vi "Keyence LJ-X8000A Driver Test.vi"() -> ()   [LabVIEW 2020]
doc: "This example mainly shows the function of each VI.\nOn each button is the name of a VI. Click a button to perform that VI."
uses:
  Public/Clusters/Read Profile Req.ctl
  Public/Constants/Profile Pos.ctl
  Public/Clusters/Read Profile Rsp.ctl
  Public/Clusters/Profile Info.ctl
  Public/Clusters/Ethernet Config.ctl
  Public/Clusters/Read Batch Profile Rsp.ctl
  Public/Clusters/Read Batch Profile Req.ctl
  Public/Constants/Batch Pos.ctl
  Public/Constants/Setting Depth.ctl
  Public/Clusters/Target Setting.ctl
  Public/Constants/Setting Type.ctl
  Public/Constants/Init Setting Target.ctl
  KEYENCE LJ-X8000A.lvlib
panel:
  out "error out":errorcluster {"code" format="%.0x"}
  in  "tab2":T1(tab)
  in  "btnTrigger":bool
  in  "btnStartMeasure":bool
  in  "btnStopMeasure":bool
  in  "btnClearMemory":bool
  out "TRG_PASS":bool
  out "MEM_FULL":bool
  out "TRG_ERROR":bool
  in  "btnGetAttentionStatus":bool
  in  "State":bool
  in  "btnControlLaser":bool
  in  "btnResetTriggerError":bool
  in  "Read Req":T2={"Read Area"=enum."ACTIVE_BANK", "Profile Pos"=0, "Read Profile No."=0, "Read Profile Cnt"=1, "isErase"=FALSE} {"Profile Pos" items=["CURRENT", "OLDEST", "SPECIFY"]}
  in  "btnReadProfiles":bool
  in  "Data Size (0: Auto Size)":u32
  out "Profile Rsp":T4
  out "Profile Data":u32[](array[numeric])
  out "Profile Info":T5
  in  "btnReadBatchProfiles":bool
  out "Batch Profile Data":u32[](array[numeric])
  out "Batch Profile Info":T5
  out "Read Batch Profile Rsp":T6
  in  "Read Batch Profile Req":T7={"Read Area"=enum."ACTIVE_BANK", "Batch Pos"=0, "Read Batch No"=0, "Read Profile No."=0, "Read Profile Cnt"=1, "isErase"=FALSE} {"Batch Pos" items=["CURRENT"=0, "SPECIFY"=2, "COMMITED"=3, "NEWEST PROFILE"=4]}
  in  "Data Size (0: Auto Size) 2":u32
  in  "Read Req 2":T2={"Read Area"=enum."ACTIVE_BANK", "Profile Pos"=0, "Read Profile No."=0, "Read Profile Cnt"=1, "isErase"=FALSE} {"Profile Pos" items=["CURRENT", "OLDEST", "SPECIFY"]}
  in  "btnReadProfileArray":bool
  in  "Data Size (0: Auto Size) 4":u32
  out "Profile Rsp 2":T4
  out "Profile Info 2":T5
  out "Header Array":u32[][](array[numeric])
  out "Height Profile Array":dbl[][](array[numeric])
  out "Luminance Profile Array":u16[][](array[numeric])
  in  "btnReboot":bool
  in  "btnFactorySetting":bool
  in  "btnGetHeadTemperature":bool
  in  "btnGetSerialNo":bool
  out "Controller Serial No.":string
  out "Head Serial No.":string
  in  "btnGetSystemError":bool
  in  "Get Code Cnt":u8=1
  in  "btnGetTriggerAndPulseCnt":bool
  out "Trigger Count":u32
  out "Encoder Count":i32
  out "Error Code":u16[](array[numeric]) format="%04x"
  out "Sensor Temperature":i16
  out "Processor Temperature":i16
  out "Case Temperature":i16
  in  "btnClearSystemError":bool
  out "Error Cnt":u8
  in  "Cleared Error Code":u16 format="%04x"
  out "Memory Accessing":bool
  out "Memory Accessing":bool
  in  "Target Setting":T9={"Type"=16, "Category"=0, "Item"=2, "Target 1"=0, "Target 2"=0, "Target 3"=0, "Target 4"=0} {"Target 4" format="%.0x"; "Target 3" format="%.0x"; "Target 2" format="%.0x"; "Target 1" format="%.0x"; "Item" format="%.0x"; "Category" format="%.0x"; "Type" items=["ENVIRONMENT"=1, "COMMON MEASUREMENT"=2, "PROGRAM 0"=16, "PROGRAM 1"=17, "PROGRAM 2"=18, "PROGRAM 3"=19, "PROGRAM 4"=20, "PROGRAM 5"=21, "PROGRAM 6"=22, "PROGRAM 7"=23, "PROGRAM 8"=24, "PROGRAM 9"=25, "PROGRAM 10"=26, "PROGRAM 11"=27, "PROGRAM 12"=28, "PROGRAM 13"=29, "PROGRAM 14"=30, "PROGRAM 15"=31]}
  in  "Depth":T11=1 items=["WRITE AREA", "RUNNING AREA", "SAVE AREA"]
  in  "btnChangeProgram":bool
  in  "btnGetProgram":bool
  in  "Program No":u8
  out "Active Program No.":u8
  in  "Target Setting":T9={"Type"=16, "Category"=0, "Item"=2, "Target 1"=0, "Target 2"=0, "Target 3"=0, "Target 4"=0} {"Target 4" format="%.0x"; "Target 3" format="%.0x"; "Target 2" format="%.0x"; "Target 1" format="%.0x"; "Item" format="%.0x"; "Category" format="%.0x"; "Type" items=["ENVIRONMENT"=1, "COMMON MEASUREMENT"=2, "PROGRAM 0"=16, "PROGRAM 1"=17, "PROGRAM 2"=18, "PROGRAM 3"=19, "PROGRAM 4"=20, "PROGRAM 5"=21, "PROGRAM 6"=22, "PROGRAM 7"=23, "PROGRAM 8"=24, "PROGRAM 9"=25, "PROGRAM 10"=26, "PROGRAM 11"=27, "PROGRAM 12"=28, "PROGRAM 13"=29, "PROGRAM 14"=30, "PROGRAM 15"=31]}
  out "Setting Data":u8[](array[numeric])
  in  "Depth":T11=1 items=["WRITE AREA", "RUNNING AREA", "SAVE AREA"]
  in  "btnGetSetting":bool
  in  "Data Size":u32=4
  in  "btnSetSetting":bool
  in  "Setting Data":u8[](array[numeric])=[3, 0, 0, 0]
  out "Setting Error":u32 format="%.0x"
  out "Memory Accessing":bool
  in  "Depth":T11 items=["WRITE AREA", "RUNNING AREA", "SAVE AREA"]
  in  "btnInitializeSetting":bool
  in  "Target Program":T12 items=["PROGRAM 0", "PROGRAM 1", "PROGRAM 2", "PROGRAM 3", "PROGRAM 4", "PROGRAM 5", "PROGRAM 6", "PROGRAM 7", "PROGRAM 8", "PROGRAM 9", "PROGRAM 10", "PROGRAM 11", "PROGRAM 12", "PROGRAM 13", "PROGRAM 14", "PROGRAM 15"]
  in  "Depth":T11 items=["WRITE AREA", "RUNNING AREA", "SAVE AREA"]
  in  "btnReflectSetting":bool
  out "Setting Error":u32
  in  "btnUpdateWriteSettingArea":bool
  in  "Depth":T11 items=["WRITE AREA", "RUNNING AREA", "SAVE AREA"]
  in  "btnLogClear":bool
  in  "btnClose":bool
  out "Operation Result Log":string
  out "isConnecting":bool caption="Connecting"
  in  "Ethernet Config":T13={"IP Address"=[192, 168, 0, 1], "Port No"=24691}
  in  "btnInitialize":bool
  in  "stop":bool caption="’âŽ~"
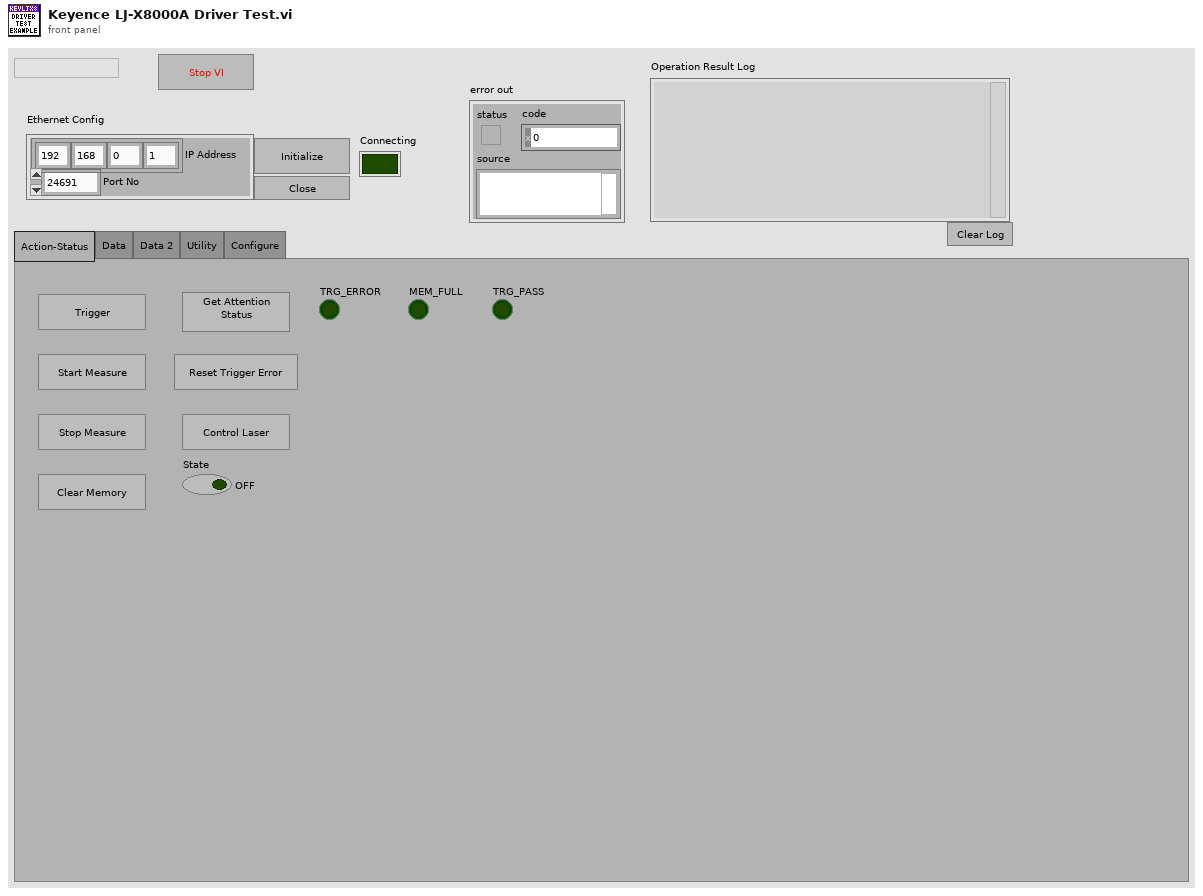
[diagram p1: front panel]
types:
  T1 = enum32{"Action-Status", "Data", "Data 2", "Utility", "Configure"}
  T2 = typedef "KEYENCE LJ-X8000A.lvlib/Read Profile Req.ctl" = cluster{"Read Area":enum8{"ACTIVE_BANK", "INACTIVE_BANK"}, "Profile Pos":T3, "Read Profile No.":u32, "Read Profile Cnt":u8, "isErase":bool}
  T3 = typedef "KEYENCE LJ-X8000A.lvlib/Profile Pos.ctl" = u8
  T4 = typedef "KEYENCE LJ-X8000A.lvlib/Read Profile Rsp.ctl" = cluster{"Current Profile No":u32, "Oldest Profile No":u32, "Read Top Profile No":u32, "Read Profile Cnt":u8}
  T5 = typedef "KEYENCE LJ-X8000A.lvlib/Profile Info.ctl" = cluster{"Profile Cnt":u8, "Luminance Output":bool, " Profile Data Point":u16, " X Start":i32, " X Pitch":i32}
  T6 = typedef "KEYENCE LJ-X8000A.lvlib/Read Batch Profile Rsp.ctl" = cluster{"Current Batch No":u32, "Current Batch Profile Cnt":u32, "Oldest Batch No":u32, "Oldest Batch Profile Cnt":u32, "Read Batch No":u32, "Read Batch Profile Cnt":u32, "Read Batch Top Profile No":u32, "Read Profile Cnt":u32, "Current Batch Commited":bool}
  T7 = typedef "KEYENCE LJ-X8000A.lvlib/Read Batch Profile Req.ctl" = cluster{"Read Area":enum8{"ACTIVE_BANK", "INACTIVE_BANK"}, "Batch Pos":T8, "Read Batch No":u32, "Read Profile No.":u32, "Read Profile Cnt":u8, "isErase":bool}
  T8 = typedef "KEYENCE LJ-X8000A.lvlib/Batch Pos.ctl" = u8
  T9 = typedef "KEYENCE LJ-X8000A.lvlib/Target Setting.ctl" = cluster{"Type":T10, "Category":u8, "Item":u8, "Target 1":u8, "Target 2":u8, "Target 3":u8, "Target 4":u8}
  T10 = typedef "KEYENCE LJ-X8000A.lvlib/Setting Type.ctl" = u8
  T11 = typedef "KEYENCE LJ-X8000A.lvlib/Setting Depth.ctl" = u8
  T12 = typedef "KEYENCE LJ-X8000A.lvlib/Init Setting Target.ctl" = u8
  T13 = typedef "KEYENCE LJ-X8000A.lvlib/Ethernet Config.ctl" = cluster{"IP Address":u8[], "Port No":u16}
  T14 = enum8{"Enabled", "Disabled", "Disabled and Grayed Out"}
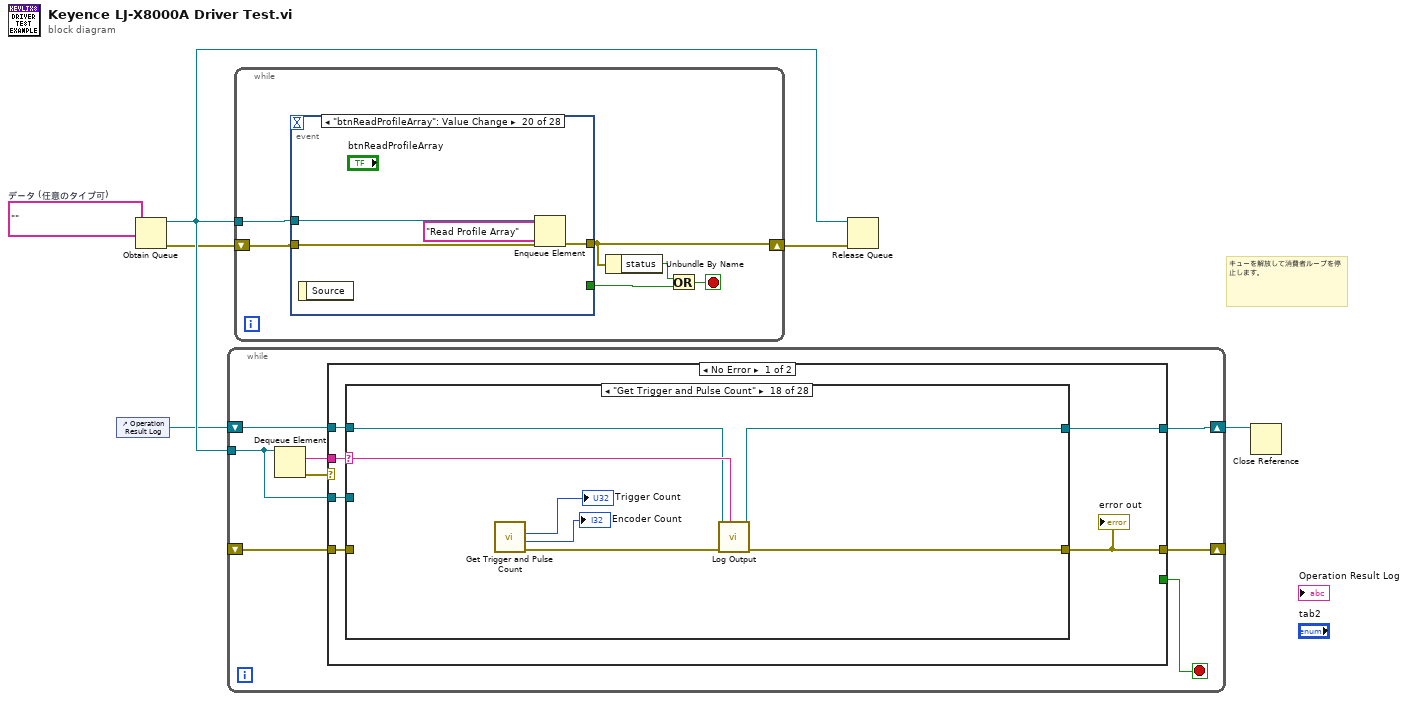
[diagram p0: block diagram]
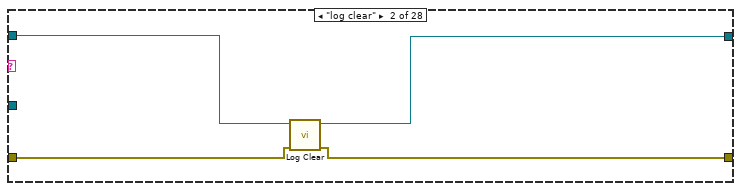
[diagram p3: hidden frame]
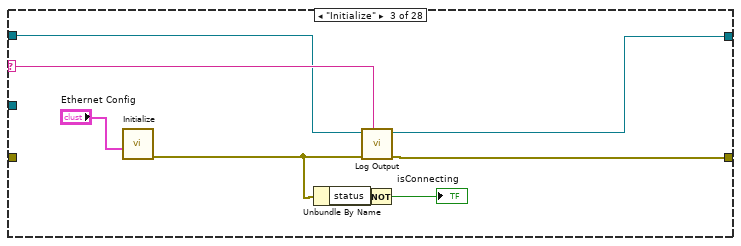
[diagram p4: hidden frame]
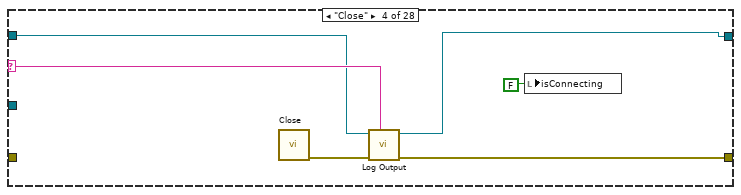
[diagram p5: hidden frame]
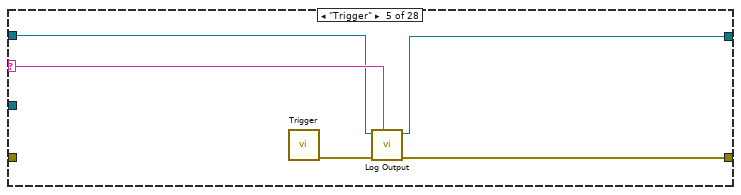
[diagram p6: hidden frame]
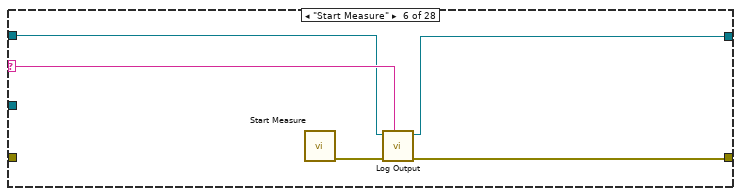
[diagram p7: hidden frame]
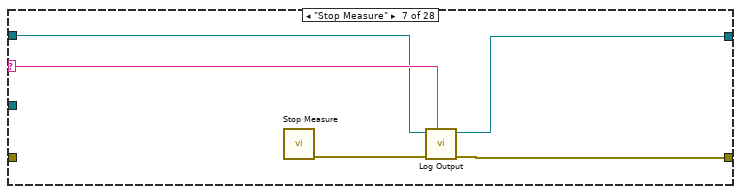
[diagram p8: hidden frame]
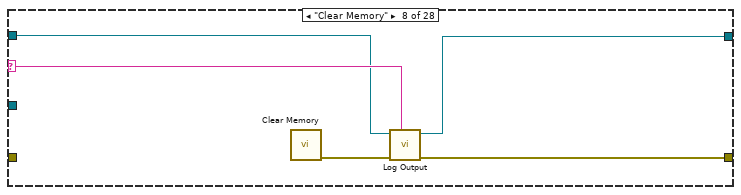
[diagram p9: hidden frame]
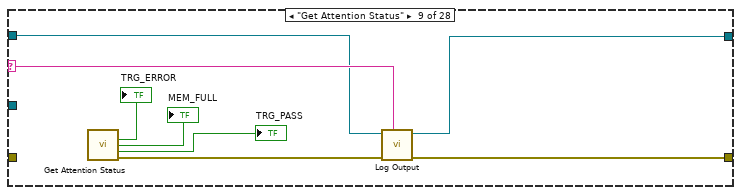
[diagram p10: hidden frame]
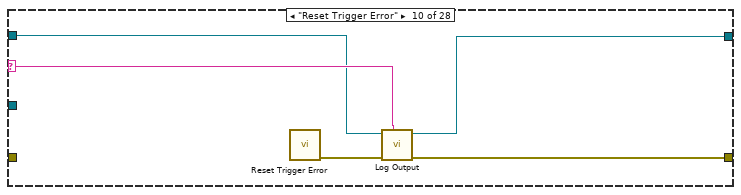
[diagram p11: hidden frame]
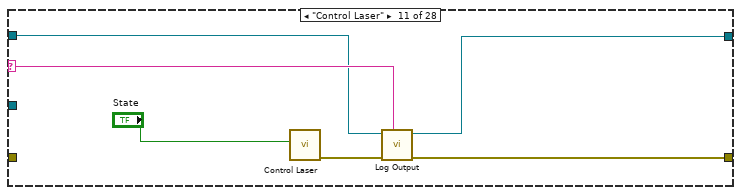
[diagram p12: hidden frame]
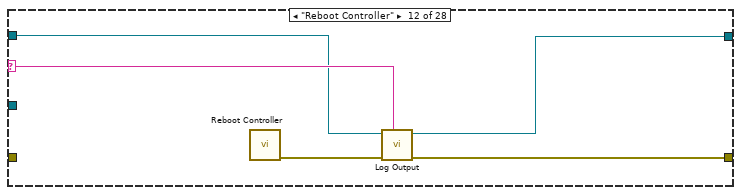
[diagram p13: hidden frame]
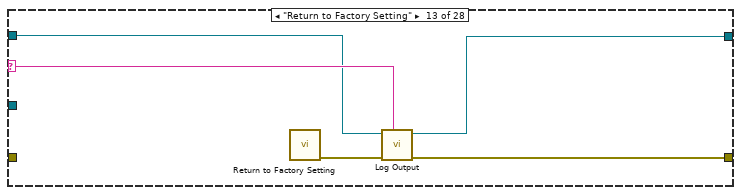
[diagram p14: hidden frame]
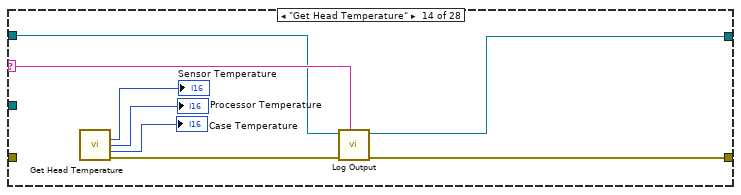
[diagram p15: hidden frame]
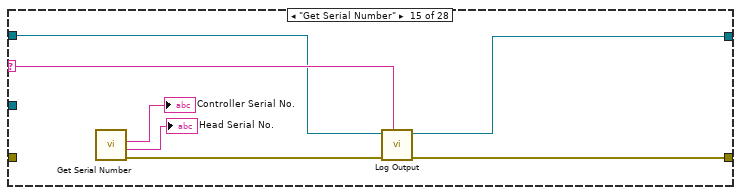
[diagram p16: hidden frame]
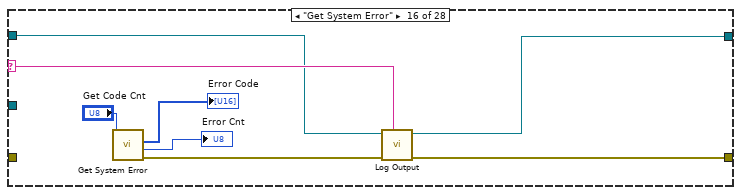
[diagram p17: hidden frame]
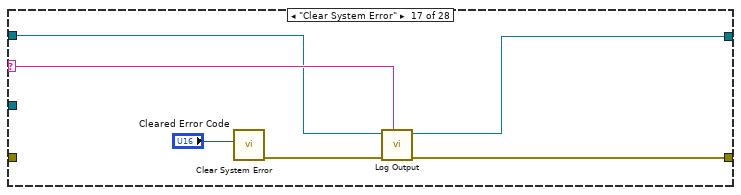
[diagram p18: hidden frame]
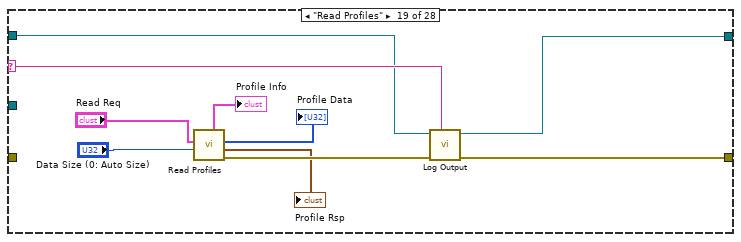
[diagram p19: hidden frame]
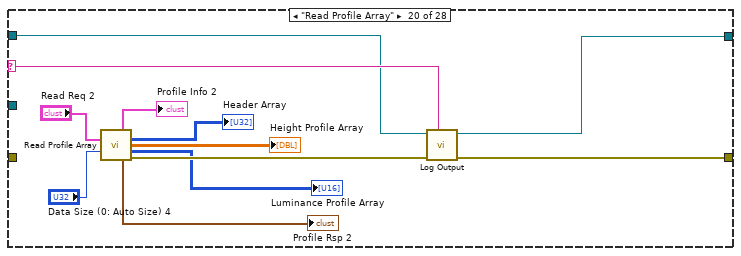
[diagram p20: hidden frame]
diagram:
  w6 = ""  # データ (任意のタイプ可)
  # "キューを解放して消費者ループを停止します。"
  n1 = control-ref of="Operation Result Log"() -> (w2:refnum<vi>)
  n2 = Obtain Queue(element data type=w6) -> (queue out=w5:refnum<queue>, error out=w3:errorcluster)  [unwired: 4 in, 1 out]
  n3 = while {
    tunnel: w5 -> [w10]
    shift-right: [w9] -> _
    shift-left: _ -> [w11]
    shift-right: [w7] -> w1
    shift-left: w2 -> [w8]
    stop <- w12 stop-if-true
    n4 = Dequeue Element(queue=w10) -> (element=w13:string, error out=w14:errorcluster)  [unwired: 2 in, 2 out]
    n5 = case shown="No Error" w14 {
      selector: w14 -> [_ w243]
      tunnel: w13 -> [w20 _]
      tunnel: [_ TRUE] -> w12
      tunnel: [w19 w243] -> w9
      tunnel: w11 -> [w18 _]
      tunnel: w10 -> [w17 _]
      tunnel: w8 -> [w15 w241]
      tunnel: [w16 w241] -> w7
      frame No Error {
        n6 = case shown="\"Get Trigger and Pulse Count\"" w20 {
          selector: w20 -> [_ _ w29 w37 w43 w48 w53 w58 w63 w71 w76 w82 w87 w92 w100 w107 w115 w121 w128 w146 w150 w160 w166 w172 w181 w203 w222 w237]
          tunnel: [w22 w24 w30 w38 w44 w49 w54 w59 w68 w73 w79 w84 w89 w97 w104 w112 w118 w125 w135 w147 w157 w163 w169 w178 w184 w201 w219 w240] -> w19
          tunnel: w18 -> [w22 w25 _ _ _ _ _ _ _ _ _ _ _ _ _ _ _ _ _ _ _ _ _ _ _ _ _ _]
          tunnel: w17 -> [_ _ _ _ _ _ _ _ _ _ _ _ _ _ _ _ _ _ _ _ _ _ _ _ _ _ _ _]
          tunnel: w15 -> [w21 w26 w28 w36 w42 w47 w52 w57 w62 w70 w75 w81 w86 w91 w99 w106 w114 w120 w127 w137 w149 w159 w165 w170 w180 w200 w218 w236]
          tunnel: [w21 w23 w27 w35 w41 w46 w51 w56 w61 w69 w74 w80 w85 w90 w98 w105 w113 w119 w126 w136 w148 w158 w164 w171 w179 w199 w217 w235] -> w16
          frame Default {
          }
          frame "log clear" {
            n7 = call "Log Clear.vi"("error in (no error)"=w25, "Result Log Reference"=w26) -> ("error out"=w24:errorcluster, "Result Log Reference Out"=w23:refnum<vi>)  [unwired: 8 in]
          }
          frame "Initialize" {
            n8 = call "Initialize.vi"("Ethernet Config"="Ethernet Config") -> ("error out"=w31:errorcluster)  [unwired: 9 in, 1 out]
            n9 = Unbundle By Name(w31) -> ("status"=w33:bool)
            n10 = call "Log Output.vi"("VI Name"=w29, "error in (no error)"=w31, "Result Log Reference"=w28) -> ("error out"=w30:errorcluster, "Result Log Reference Out"=w27:refnum<vi>)  [unwired: 6 in]
            n11 = Not(x=w33) -> (.not. x?=→"isConnecting":bool)
          }
          frame "Close" {
            n12 = call "Close.vi"() -> ("error out"=w39:errorcluster)  [unwired: 10 in, 1 out]
            n13 = call "Log Output.vi"("VI Name"=w37, "error in (no error)"=w39, "Result Log Reference"=w36) -> ("error out"=w38:errorcluster, "Result Log Reference Out"=w35:refnum<vi>)  [unwired: 6 in]
            n14 = local write "isConnecting"(FALSE ("isConnecting")) -> ()
          }
          frame "Trigger" {
            n15 = call "Trigger.vi"() -> ("error out"=w45:errorcluster)  [unwired: 10 in, 1 out]
            n16 = call "Log Output.vi"("VI Name"=w43, "error in (no error)"=w45, "Result Log Reference"=w42) -> ("error out"=w44:errorcluster, "Result Log Reference Out"=w41:refnum<vi>)  [unwired: 6 in]
          }
          frame "Start Measure" {
            n17 = call "Start Measure.vi"() -> ("error out"=w50:errorcluster)  [unwired: 10 in, 1 out]
            n18 = call "Log Output.vi"("VI Name"=w48, "error in (no error)"=w50, "Result Log Reference"=w47) -> ("error out"=w49:errorcluster, "Result Log Reference Out"=w46:refnum<vi>)  [unwired: 6 in]
          }
          frame "Stop Measure" {
            n19 = call "Stop Measure.vi"() -> ("error out"=w55:errorcluster)  [unwired: 10 in, 1 out]
            n20 = call "Log Output.vi"("VI Name"=w53, "error in (no error)"=w55, "Result Log Reference"=w52) -> ("error out"=w54:errorcluster, "Result Log Reference Out"=w51:refnum<vi>)  [unwired: 6 in]
          }
          frame "Clear Memory" {
            n21 = call "Clear Memory.vi"() -> ("error out"=w60:errorcluster)  [unwired: 10 in, 1 out]
            n22 = call "Log Output.vi"("VI Name"=w58, "error in (no error)"=w60, "Result Log Reference"=w57) -> ("error out"=w59:errorcluster, "Result Log Reference Out"=w56:refnum<vi>)  [unwired: 6 in]
          }
          frame "Get Attention Status" {
            n23 = call "Get Attention Status.vi"() -> ("TRG_ERROR"=→"TRG_ERROR":bool, "MEM_FULL"=→"MEM_FULL":bool, "TRG_PASS"=→"TRG_PASS":bool, "error out"=w67:errorcluster)  [unwired: 11 in, 1 out]
            n24 = call "Log Output.vi"("VI Name"=w63, "error in (no error)"=w67, "Result Log Reference"=w62) -> ("error out"=w68:errorcluster, "Result Log Reference Out"=w61:refnum<vi>)  [unwired: 6 in]
          }
          frame "Reset Trigger Error" {
            n25 = call "Reset Trigger Error.vi"() -> ("error out"=w72:errorcluster)  [unwired: 10 in, 1 out]
            n26 = call "Log Output.vi"("VI Name"=w71, "error in (no error)"=w72, "Result Log Reference"=w70) -> ("error out"=w73:errorcluster, "Result Log Reference Out"=w69:refnum<vi>)  [unwired: 6 in]
          }
          frame "Control Laser" {
            n27 = call "Control Laser.vi"("State"="State") -> ("error out"=w78:errorcluster)  [unwired: 9 in, 1 out]
            n28 = call "Log Output.vi"("VI Name"=w76, "error in (no error)"=w78, "Result Log Reference"=w75) -> ("error out"=w79:errorcluster, "Result Log Reference Out"=w74:refnum<vi>)  [unwired: 6 in]
          }
          frame "Reboot Controller" {
            n29 = call "Reboot Controller.vi"() -> ("error out"=w83:errorcluster)  [unwired: 10 in, 1 out]
            n30 = call "Log Output.vi"("VI Name"=w82, "error in (no error)"=w83, "Result Log Reference"=w81) -> ("error out"=w84:errorcluster, "Result Log Reference Out"=w80:refnum<vi>)  [unwired: 6 in]
          }
          frame "Return to Factory Setting" {
            n31 = call "Return to Factory Setting.vi"() -> ("error out"=w88:errorcluster)  [unwired: 10 in, 1 out]
            n32 = call "Log Output.vi"("VI Name"=w87, "error in (no error)"=w88, "Result Log Reference"=w86) -> ("error out"=w89:errorcluster, "Result Log Reference Out"=w85:refnum<vi>)  [unwired: 6 in]
          }
          frame "Get Head Temperature" {
            n33 = call "Get Head Temperature.vi"() -> ("Sensor Temperature"=→"Sensor Temperature":i16, "Processor Temperature"=→"Processor Temperature":i16, "Case Temperature"=→"Case Temperature":i16, "error out"=w96:errorcluster)  [unwired: 11 in, 1 out]
            n34 = call "Log Output.vi"("VI Name"=w92, "error in (no error)"=w96, "Result Log Reference"=w91) -> ("error out"=w97:errorcluster, "Result Log Reference Out"=w90:refnum<vi>)  [unwired: 6 in]
          }
          frame "Get Serial Number" {
            n35 = call "Get Serial Number.vi"() -> ("error out"=w103:errorcluster, "Head Serial No."=→"Head Serial No.":string, "Controller Serial No."=→"Controller Serial No.":string)  [unwired: 8 in, 1 out]
            n36 = call "Log Output.vi"("VI Name"=w100, "error in (no error)"=w103, "Result Log Reference"=w99) -> ("error out"=w104:errorcluster, "Result Log Reference Out"=w98:refnum<vi>)  [unwired: 6 in]
          }
          frame "Get System Error" {
            n37 = call "Get System Error.vi"("Get Code Cnt"="Get Code Cnt") -> ("error out"=w111:errorcluster, "Error Cnt"=→"Error Cnt":u8, "Error Code"=→"Error Code":u16[])  [unwired: 7 in, 1 out]
            n38 = call "Log Output.vi"("VI Name"=w107, "error in (no error)"=w111, "Result Log Reference"=w106) -> ("error out"=w112:errorcluster, "Result Log Reference Out"=w105:refnum<vi>)  [unwired: 6 in]
          }
          frame "Clear System Error" {
            n39 = call "Clear System Error.vi"("Error Code"="Cleared Error Code") -> ("error out"=w117:errorcluster)  [unwired: 9 in, 1 out]
            n40 = call "Log Output.vi"("VI Name"=w115, "error in (no error)"=w117, "Result Log Reference"=w114) -> ("error out"=w118:errorcluster, "Result Log Reference Out"=w113:refnum<vi>)  [unwired: 6 in]
          }
          frame "Get Trigger and Pulse Count" {
            n41 = call "Get Trigger and Pulse Count.vi"() -> ("error out"=w124:errorcluster, "Encoder Count"=→"Encoder Count":i32, "Trigger Count"=→"Trigger Count":u32)  [unwired: 8 in, 1 out]
            n42 = call "Log Output.vi"("VI Name"=w121, "error in (no error)"=w124, "Result Log Reference"=w120) -> ("error out"=w125:errorcluster, "Result Log Reference Out"=w119:refnum<vi>)  [unwired: 6 in]
          }
          frame "Read Profiles" {
            n43 = call "Read Profiles.vi"("Data Size (0: Auto Size)"="Data Size (0: Auto Size)", "Read Req"="Read Req") -> ("error out"=w134:errorcluster, "Profile Rsp"=→"Profile Rsp":T4, "Profile Data"=→"Profile Data":u32[], "Profile Info"=→"Profile Info":T5)  [unwired: 5 in, 1 out]
            n44 = call "Log Output.vi"("VI Name"=w128, "error in (no error)"=w134, "Result Log Reference"=w127) -> ("error out"=w135:errorcluster, "Result Log Reference Out"=w126:refnum<vi>)  [unwired: 6 in]
          }
          frame "Read Profile Array" {
            n45 = call "Read Profile Array.vi"("Read Req"="Read Req 2", "Data Size (0: Auto Size)"="Data Size (0: Auto Size) 4") -> ("Profile Info"=→"Profile Info 2":T5, "Header Array"=→"Header Array":u32[][], "Height Profile Array"=→"Height Profile Array":dbl[][], "Luminance Profile Array"=→"Luminance Profile Array":u16[][], "Profile Rsp"=→"Profile Rsp 2":T4, "error out"=w145:errorcluster)  [unwired: 7 in, 1 out]
            n46 = call "Log Output.vi"("VI Name"=w146, "error in (no error)"=w145, "Result Log Reference"=w137) -> ("error out"=w147:errorcluster, "Result Log Reference Out"=w136:refnum<vi>)  [unwired: 6 in]
          }
          frame "Read Batch Profiles" {
            n47 = call "Read Batch Profiles.vi"("Data Size (0: Auto Size)"="Data Size (0: Auto Size) 2", "Read Batch Profile Req"="Read Batch Profile Req") -> ("error out"=w156:errorcluster, "Read Batch Profile Rsp"=→"Read Batch Profile Rsp":T6, "Profile Data"=→"Batch Profile Data":u32[], "Profile Info"=→"Batch Profile Info":T5)  [unwired: 5 in, 1 out]
            n48 = call "Log Output.vi"("VI Name"=w150, "error in (no error)"=w156, "Result Log Reference"=w149) -> ("error out"=w157:errorcluster, "Result Log Reference Out"=w148:refnum<vi>)  [unwired: 6 in]
          }
          frame "Change Program" {
            n49 = call "Change Program.vi"("Program No"="Program No") -> ("error out"=w162:errorcluster)  [unwired: 9 in, 1 out]
            n50 = call "Log Output.vi"("VI Name"=w160, "error in (no error)"=w162, "Result Log Reference"=w159) -> ("error out"=w163:errorcluster, "Result Log Reference Out"=w158:refnum<vi>)  [unwired: 6 in]
          }
          frame "Get Active Program Number" {
            n51 = call "Get Active Program Number.vi"() -> ("error out"=w168:errorcluster, "Program No"=→"Active Program No.":u8)  [unwired: 9 in, 1 out]
            n52 = call "Log Output.vi"("VI Name"=w166, "error in (no error)"=w168, "Result Log Reference"=w165) -> ("error out"=w169:errorcluster, "Result Log Reference Out"=w164:refnum<vi>)  [unwired: 6 in]
          }
          frame "Get Setting" {
            n53 = call "Get Setting.vi"("Depth"="Depth", "Data Size"="Data Size", "Target Setting"="Target Setting") -> ("error out"=w177:errorcluster, "Setting Data"=→"Setting Data":u8[])  [unwired: 6 in, 1 out]
            n54 = call "Log Output.vi"("VI Name"=w172, "error in (no error)"=w177, "Result Log Reference"=w170) -> ("error out"=w178:errorcluster, "Result Log Reference Out"=w171:refnum<vi>)  [unwired: 6 in]
          }
          frame "Set Setting" {
            n55 = call "Set Setting.vi"("Depth"="Depth", "Setting Data"="Setting Data", "Target Setting"="Target Setting") -> ("error out"=w183:errorcluster, "Setting Error"=→"Setting Error":u32)  [unwired: 6 in, 1 out]
            n56 = call "Log Output.vi"("VI Name"=w181, "error in (no error)"=w183, "Result Log Reference"=w180) -> ("error out"=w182:errorcluster, "Result Log Reference Out"=w179:refnum<vi>)  [unwired: 6 in]
            n57 = while {
              tunnel: w182 -> [w198]
              tunnel: [w197] -> w185
              stop <- w195 stop-if-true
              n58 = call "Check Status of Saving to Save Area.vi"("error in (no error)"=w198) -> ("error out"=w197:errorcluster, "Busy"=w193:bool)  [unwired: 8 in, 1 out]
              "Memory Accessing" <- w193
              n59 = Not(x=w193) -> (.not. x?=w194:bool)
              n60 = Unbundle By Name(w197) -> ("status"=w192:bool)
              n61 = Or(x=w194, y=w192) -> (x .or. y?=w195:bool)
              n62 = Wait Until Next ms Multiple(millisecond multiple=u32 100 ("ミリ秒倍数")) -> ()  [unwired: 1 out]
            }
            n63 = flat-sequence {
              tunnel: w185 -> [w190]
              tunnel: [w190] -> w184
              frame #0 {
                n64 = property on="btnSetSetting" class="Bool"("DisabledEnum"=T14."Enabled" ("–³Œø")) -> ()  [unwired: 2 in, 2 out]
              }
            }
          }
          frame "Initialize Setting" {
            n65 = call "Initialize Setting.vi"("Depth"="Depth", "Target"="Target Program") -> ("error out"=w207:errorcluster)  [unwired: 8 in, 1 out]
            n66 = call "Log Output.vi"("VI Name"=w203, "error in (no error)"=w207, "Result Log Reference"=w200) -> ("error out"=w204:errorcluster, "Result Log Reference Out"=w199:refnum<vi>)  [unwired: 6 in]
            n67 = while {
              tunnel: w204 -> [w216]
              tunnel: [w215] -> w202
              stop <- w213 stop-if-true
              n68 = call "Check Status of Saving to Save Area.vi"("error in (no error)"=w216) -> ("error out"=w215:errorcluster, "Busy"=w211:bool)  [unwired: 8 in, 1 out]
              "Memory Accessing" <- w211
              n69 = Not(x=w211) -> (.not. x?=w212:bool)
              n70 = Unbundle By Name(w215) -> ("status"=w210:bool)
              n71 = Or(x=w212, y=w210) -> (x .or. y?=w213:bool)
              n72 = Wait Until Next ms Multiple(millisecond multiple=u32 100 ("ミリ秒倍数")) -> ()  [unwired: 1 out]
            }
            n73 = flat-sequence {
              tunnel: w202 -> [w209]
              tunnel: [w209] -> w201
              frame #0 {
                n74 = property on="btnInitializeSetting" class="Bool"("DisabledEnum"=T14."Enabled" ("–³Œø")) -> ()  [unwired: 2 in, 2 out]
              }
            }
          }
          frame "Reflect Setting" {
            n75 = call "Reflect Setting.vi"("Depth"="Depth") -> ("error out"=w225:errorcluster, "Setting Error"=→"Setting Error":u32)  [unwired: 8 in, 1 out]
            n76 = call "Log Output.vi"("VI Name"=w222, "error in (no error)"=w225, "Result Log Reference"=w218) -> ("error out"=w221:errorcluster, "Result Log Reference Out"=w217:refnum<vi>)  [unwired: 6 in]
            n77 = while {
              tunnel: w221 -> [w232]
              tunnel: [w231] -> w220
              stop <- w229 stop-if-true
              n78 = call "Check Status of Saving to Save Area.vi"("error in (no error)"=w232) -> ("error out"=w231:errorcluster, "Busy"=w227:bool)  [unwired: 8 in, 1 out]
              "Memory Accessing" <- w227
              n79 = Not(x=w227) -> (.not. x?=w228:bool)
              n80 = Unbundle By Name(w231) -> ("status"=w226:bool)
              n81 = Or(x=w228, y=w226) -> (x .or. y?=w229:bool)
              n82 = Wait Until Next ms Multiple(millisecond multiple=u32 100 ("ミリ秒倍数")) -> ()  [unwired: 1 out]
            }
            n83 = flat-sequence {
              tunnel: w220 -> [w233]
              tunnel: [w233] -> w219
              frame #0 {
                n84 = property on="btnReflectSetting" class="Bool"("DisabledEnum"=T14."Enabled" ("–³Œø")) -> ()  [unwired: 2 in, 2 out]
              }
            }
          }
          frame "Update Write Setting Area" {
            n85 = call "Update Write Setting Area.vi"("Depth"="Depth") -> ("error out"=w239:errorcluster)  [unwired: 9 in, 1 out]
            n86 = call "Log Output.vi"("VI Name"=w237, "error in (no error)"=w239, "Result Log Reference"=w236) -> ("error out"=w240:errorcluster, "Result Log Reference Out"=w235:refnum<vi>)  [unwired: 6 in]
          }
        }
        "error out" <- w19
      }
      frame Error {
        n87 = call "Close.vi"() -> ()  [unwired: 10 in, 2 out]
        n88 = local write "isConnecting"(FALSE ("isConnecting")) -> ()
      }
    }
  }
  n89 = while {
    shift-right: [w246] -> w4
    shift-left: w3 -> [w249]
    tunnel: w5 -> [w250]
    stop <- w247 stop-if-true
    n90 = event shown="[19] \"btnReadProfileArray\": Value Change" {
      selector: _ -> [_ _ _ _ _ _ _ _ _ _ _ _ _ _ _ _ _ _ _ _ _ _ _ _ _ _ _ _]
      dyn-events: _ -> [_ _ _ _ _ _ _ _ _ _ _ _ _ _ _ _ _ _ _ _ _ _ _ _ _ _ _ _]
      timeout: _ -> [_ _ _ _ _ _ _ _ _ _ _ _ _ _ _ _ _ _ _ _ _ _ _ _ _ _ _ _]
      tunnel: w250 -> [_ w254 w260 w264 w268 w272 w276 w280 w284 w288 w292 w296 w300 w304 w308 w312 w316 w320 w324 w328 w332 w336 w340 w344 w349 w354 w359 w363]
      tunnel: w249 -> [w251 w256 w259 w263 w267 w271 w275 w279 w283 w287 w291 w295 w299 w303 w307 w311 w315 w319 w323 w327 w331 w335 w339 w343 w348 w353 w358 w362]
      tunnel: [w251 w255 w258 w262 w266 w270 w274 w278 w282 w286 w290 w294 w298 w302 w306 w310 w314 w318 w322 w326 w330 w334 w338 w342 w347 w352 w357 w361] -> w246
      tunnel: ["stop" _ _ _ _ _ _ _ _ _ _ _ _ _ _ _ _ _ _ _ _ _ _ _ _ _ _ _] -> w248
      event "stop": Value Change {
        n91 = event-data() -> ()  [unwired: 1 in, 1 out]
      }
      event "btnLogClear": Value Change {
        n92 = event-data() -> ()  [unwired: 1 in, 1 out]
        n93 = Enqueue Element(queue=w254, element="log clear", error in (no error)=w256) -> (error out=w255:errorcluster)  [unwired: 1 in, 2 out]
      }
      event "btnInitialize": Value Change {
        n94 = event-data() -> ()  [unwired: 1 in, 1 out]
        n95 = Enqueue Element(queue=w260, element="Initialize", error in (no error)=w259) -> (error out=w258:errorcluster)  [unwired: 1 in, 2 out]
      }
      event "btnClose": Value Change {
        n96 = event-data() -> ()  [unwired: 1 in, 1 out]
        n97 = Enqueue Element(queue=w264, element="Close", error in (no error)=w263) -> (error out=w262:errorcluster)  [unwired: 1 in, 2 out]
      }
      event "btnTrigger": Value Change {
        n98 = event-data() -> ()  [unwired: 1 in, 1 out]
        n99 = Enqueue Element(queue=w268, element="Trigger", error in (no error)=w267) -> (error out=w266:errorcluster)  [unwired: 1 in, 2 out]
      }
      event "btnStartMeasure": Value Change {
        n100 = event-data() -> ()  [unwired: 1 in, 1 out]
        n101 = Enqueue Element(queue=w272, element="Start Measure", error in (no error)=w271) -> (error out=w270:errorcluster)  [unwired: 1 in, 2 out]
      }
      event "btnStopMeasure": Value Change {
        n102 = event-data() -> ()  [unwired: 1 in, 1 out]
        n103 = Enqueue Element(queue=w276, element="Stop Measure", error in (no error)=w275) -> (error out=w274:errorcluster)  [unwired: 1 in, 2 out]
      }
      event "btnClearMemory": Value Change {
        n104 = event-data() -> ()  [unwired: 1 in, 1 out]
        n105 = Enqueue Element(queue=w280, element="Clear Memory", error in (no error)=w279) -> (error out=w278:errorcluster)  [unwired: 1 in, 2 out]
      }
      event "btnReboot": Value Change {
        n106 = event-data() -> ()  [unwired: 1 in, 1 out]
        n107 = Enqueue Element(queue=w284, element="Reboot Controller", error in (no error)=w283) -> (error out=w282:errorcluster)  [unwired: 1 in, 2 out]
      }
      event "btnFactorySetting": Value Change {
        n108 = event-data() -> ()  [unwired: 1 in, 1 out]
        n109 = Enqueue Element(queue=w288, element="Return to Factory Setting", error in (no error)=w287) -> (error out=w286:errorcluster)  [unwired: 1 in, 2 out]
      }
      event "btnGetHeadTemperature": Value Change {
        n110 = event-data() -> ()  [unwired: 1 in, 1 out]
        n111 = Enqueue Element(queue=w292, element="Get Head Temperature", error in (no error)=w291) -> (error out=w290:errorcluster)  [unwired: 1 in, 2 out]
      }
      event "btnGetSerialNo": Value Change {
        n112 = event-data() -> ()  [unwired: 1 in, 1 out]
        n113 = Enqueue Element(queue=w296, element="Get Serial Number", error in (no error)=w295) -> (error out=w294:errorcluster)  [unwired: 1 in, 2 out]
      }
      event "btnGetSystemError": Value Change {
        n114 = event-data() -> ()  [unwired: 1 in, 1 out]
        n115 = Enqueue Element(queue=w300, element="Get System Error", error in (no error)=w299) -> (error out=w298:errorcluster)  [unwired: 1 in, 2 out]
      }
      event "btnClearSystemError": Value Change {
        n116 = event-data() -> ()  [unwired: 1 in, 1 out]
        n117 = Enqueue Element(queue=w304, element="Clear System Error", error in (no error)=w303) -> (error out=w302:errorcluster)  [unwired: 1 in, 2 out]
      }
      event "btnGetTriggerAndPulseCnt": Value Change {
        n118 = event-data() -> ()  [unwired: 1 in, 1 out]
        n119 = Enqueue Element(queue=w308, element="Get Trigger and Pulse Count", error in (no error)=w307) -> (error out=w306:errorcluster)  [unwired: 1 in, 2 out]
      }
      event "btnGetAttentionStatus": Value Change {
        n120 = event-data() -> ()  [unwired: 1 in, 1 out]
        n121 = Enqueue Element(queue=w312, element="Get Attention Status", error in (no error)=w311) -> (error out=w310:errorcluster)  [unwired: 1 in, 2 out]
      }
      event "btnResetTriggerError": Value Change {
        n122 = event-data() -> ()  [unwired: 1 in, 1 out]
        n123 = Enqueue Element(queue=w316, element="Reset Trigger Error", error in (no error)=w315) -> (error out=w314:errorcluster)  [unwired: 1 in, 2 out]
      }
      event "btnControlLaser": Value Change {
        n124 = event-data() -> ()  [unwired: 1 in, 1 out]
        n125 = Enqueue Element(queue=w320, element="Control Laser", error in (no error)=w319) -> (error out=w318:errorcluster)  [unwired: 1 in, 2 out]
      }
      event "btnReadProfiles": Value Change {
        n126 = event-data() -> ()  [unwired: 1 in, 1 out]
        n127 = Enqueue Element(queue=w324, element="Read Profiles", error in (no error)=w323) -> (error out=w322:errorcluster)  [unwired: 1 in, 2 out]
      }
      event "btnReadProfileArray": Value Change {
        n128 = event-data() -> ()  [unwired: 1 in, 1 out]
        n129 = Enqueue Element(queue=w328, element="Read Profile Array", error in (no error)=w327) -> (error out=w326:errorcluster)  [unwired: 1 in, 2 out]
      }
      event "btnReadBatchProfiles": Value Change {
        n130 = event-data() -> ()  [unwired: 1 in, 1 out]
        n131 = Enqueue Element(queue=w332, element="Read Batch Profiles", error in (no error)=w331) -> (error out=w330:errorcluster)  [unwired: 1 in, 2 out]
      }
      event "btnChangeProgram": Value Change {
        n132 = event-data() -> ()  [unwired: 1 in, 1 out]
        n133 = Enqueue Element(queue=w336, element="Change Program", error in (no error)=w335) -> (error out=w334:errorcluster)  [unwired: 1 in, 2 out]
      }
      event "btnGetProgram": Value Change {
        n134 = event-data() -> ()  [unwired: 1 in, 1 out]
        n135 = Enqueue Element(queue=w340, element="Get Active Program Number", error in (no error)=w339) -> (error out=w338:errorcluster)  [unwired: 1 in, 2 out]
      }
      event "btnGetSetting": Value Change {
        n136 = event-data() -> ()  [unwired: 1 in, 1 out]
        n137 = Enqueue Element(queue=w344, element="Get Setting", error in (no error)=w343) -> (error out=w342:errorcluster)  [unwired: 1 in, 2 out]
      }
      event "btnSetSetting": Value Change {
        n138 = event-data() -> ()  [unwired: 1 in, 1 out]
        n139 = property on="btnSetSetting" class="Bool"("DisabledEnum"=T14."Disabled and Grayed Out" ("–³Œø")) -> ()  [unwired: 2 in, 2 out]
        n140 = Enqueue Element(queue=w349, element="Set Setting", error in (no error)=w348) -> (error out=w347:errorcluster)  [unwired: 1 in, 2 out]
      }
      event "btnInitializeSetting": Value Change {
        n141 = event-data() -> ()  [unwired: 1 in, 1 out]
        n142 = property on="btnInitializeSetting" class="Bool"("DisabledEnum"=T14."Disabled and Grayed Out" ("–³Œø")) -> ()  [unwired: 2 in, 2 out]
        n143 = Enqueue Element(queue=w354, element="Initialize Setting", error in (no error)=w353) -> (error out=w352:errorcluster)  [unwired: 1 in, 2 out]
      }
      event "btnReflectSetting": Value Change {
        n144 = event-data() -> ()  [unwired: 1 in, 1 out]
        n145 = property on="btnReflectSetting" class="Bool"("DisabledEnum"=T14."Disabled and Grayed Out" ("–³Œø")) -> ()  [unwired: 2 in, 2 out]
        n146 = Enqueue Element(queue=w359, element="Reflect Setting", error in (no error)=w358) -> (error out=w357:errorcluster)  [unwired: 1 in, 2 out]
      }
      event "btnUpdateWriteSettingArea": Value Change {
        n147 = event-data() -> ()  [unwired: 1 in, 1 out]
        n148 = Enqueue Element(queue=w363, element="Update Write Setting Area", error in (no error)=w362) -> (error out=w361:errorcluster)  [unwired: 1 in, 2 out]
      }
    }
    n149 = Unbundle By Name(w246) -> ("status"=w245:bool)
    n150 = Or(x=w245, y=w248) -> (x .or. y?=w247:bool)
  }
  n151 = Release Queue(queue=w5, error in (no error)=w4) -> ()  [unwired: 1 in, 3 out]
  n152 = Close Reference(reference=w1) -> ()  [unwired: 1 in, 1 out]
